vi "Tosca-Update Status.vi"(1 "StimCon":T1, 2 "NumBlocks":i32, 7 "Current Block":i32, 9 "This trial":i32, 11 "error in (no error)":errorcluster, 12 "NumTrials":i32, 13 "Control Refs":T4) -> (15 "error out":errorcluster)   [LabVIEW 2020]
uses:
  Typedefs/Tosca-Control Refs.ctl
  FSM Graph VIs/LV Source/FSM Editor/FSM Editor.xctl
  Typedefs/Tosca-SCL Element.ctl
  Typedefs/Tosca-Schedule Mode.ctl
  Typedefs/Tosca-Event Type.ctl
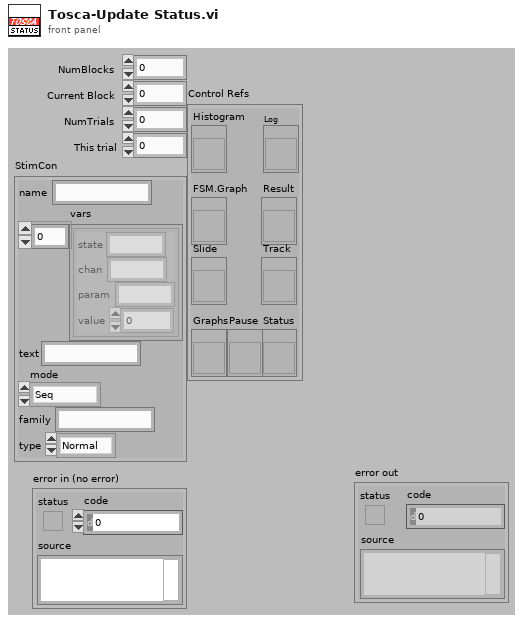
[diagram p1: front panel]
types:
  T1 = typedef "Tosca-SCL Element.ctl" = cluster{"name":string, "vars":cluster{"state":string, "chan":string, "param":string, "value":dbl}[], "text":string, "mode":T2, "family":string, "type":T3}
  T2 = typedef "Tosca-Schedule Mode.ctl" = enum16{"Seq", "CS+/CS-", "Adapt"}
  T3 = typedef "Tosca-Event Type.ctl" = enum16{"Normal", "CS+", "CS-"}
  T4 = typedef "Tosca-Control Refs.ctl" = cluster{"FSM.Graph":refnum<vi>, "Slide":refnum<vi>, "Result":refnum<vi>, "Histogram":refnum<vi>, "Graphs":refnum<vi>, "Track":refnum<vi>, "Log":refnum<vi>, "Status":refnum<vi>, "Pause":refnum<vi>}
  T5 = cluster{"state":string, "chan":string, "param":string, "value":dbl}[]
  T6 = cluster{"state":string, "chan":string, "param":string, "value":dbl}
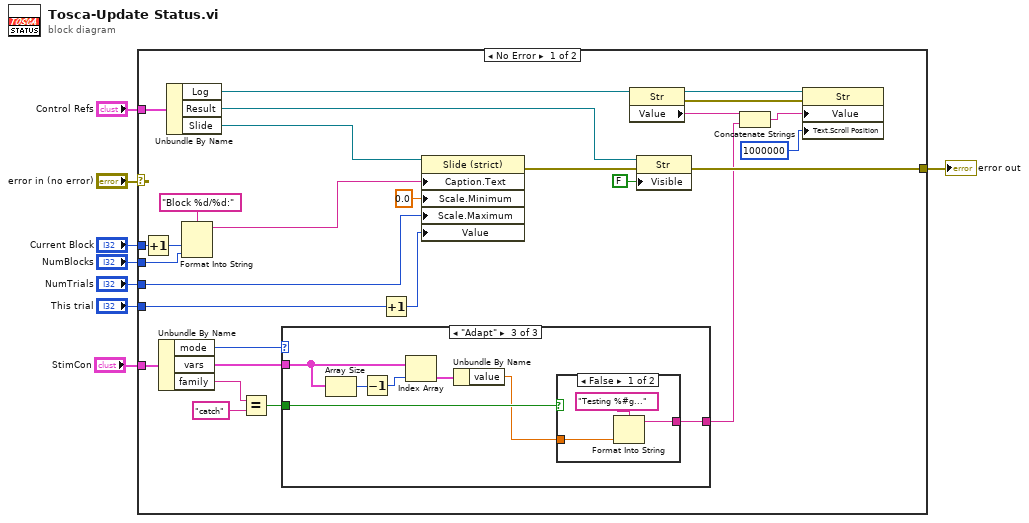
[diagram p0: block diagram]
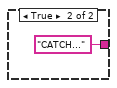
[diagram p4: hidden frame]
diagram:
  n1 = case shown="No Error" "error in (no error)" {
    selector: "error in (no error)" -> [_ w48]
    tunnel: [w26 w48] -> w7
    tunnel: "Control Refs" -> [w36 _]
    tunnel: "Current Block" -> [w33 _]
    tunnel: "NumBlocks" -> [w32 _]
    tunnel: "StimCon" -> [w13 _]
    tunnel: "NumTrials" -> [w29 _]
    tunnel: "This trial" -> [w25 _]
    frame No Error {
      n2 = Increment(x=w33) -> (x+1=w23:i32)
      n3 = Unbundle By Name(w13) -> ("mode"=w14:T2, "vars"=w9:T5, "family"=w12:string)
      n4 = Unbundle By Name(w36) -> ("Log"=w22:refnum<vi>, "Result"=w28:refnum<vi>, "Slide"=w35:refnum<vi>)
      n5 = Format Into String(format string="Block %d/%d:", w23, w32) -> (resulting string=w31:string)  [unwired: 2 in, 1 out]
      n6 = Equal?(x=w12, y="catch") -> (x = y?=w10:bool)
      n7 = case shown="\"Adapt\"" w14 {
        tunnel: [_ _ w43] -> w16
        tunnel: w10 -> [_ _ w42]
        tunnel: w9 -> [_ _ w39]
        frame "Seq", Default {
        }
        frame "CS+/CS-" {
        }
        frame "Adapt" {
          n8 = Array Size(array=w39) -> (size(s)=w38:i32)
          n9 = Decrement(x=w38) -> (x-1=w37:i32)
          n10 = Index Array(array=w39, index=w37) -> (element=w41:T6)
          n11 = Unbundle By Name(w41) -> ("value"=w40:dbl)
          n12 = case shown="False" w42 {
            tunnel: w40 -> [w45 _]
            tunnel: [w44 "CATCH..."] -> w43
            frame False {
              n13 = Format Into String(format string="Testing %#g...", w45) -> (resulting string=w44:string)  [unwired: 2 in, 1 out]
            }
            frame True {
            }
          }
        }
      }
      n14 = Increment(x=w25) -> (x+1=w24:i32)
      n15 = property class="Slide (strict)"(reference=w35, "Caption.Text"=w31, "Scale.Minimum"=0.0 ("Scale.Range:Minimum"), "Scale.Maximum"=w29, "Value"=w24) -> (error out=w15:errorcluster)  [unwired: 1 in, 1 out]
      n16 = property class="Str"(reference=w22) -> (reference out=w20:refnum<vi>, error out=w21:errorcluster, "Value"=w19:string)  [unwired: 1 in]
      n17 = property class="Str"(reference=w28, error in=w15, "Visible"=FALSE) -> (error out=w26:errorcluster)  [unwired: 1 out]
      n18 = Concatenate Strings(w19, w16) -> (w18:string)
      n19 = property class="Str"(reference=w20, error in=w21, "Value"=w18, "Text.Scroll Position"=u32 1000000) -> ()  [unwired: 2 out]
    }
    frame Error {
    }
  }
  "error out" <- w7
